vi "PH_ImageOperator.FF ConvexHull.vi"(0 "Image Src":T1, 5 "error in (no error)":errorcluster) -> (14 "Image Dst Out":T1, 19 "error out":errorcluster)   [LabVIEW 2014, in "PH_ImageOperator.lvlib"]
doc: "Calculate the convex hull of a given input image."
uses:
  PH_ImageOperator.lvlib
  <vilib>/vision/Image Controls.llb/IMAQ Image.ctl
  <vilib>/vision/NI_Vision_Development_Module.lvlib
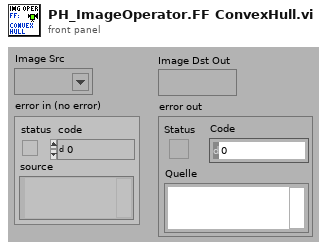
[diagram p1: front panel]
types:
  T1 = typedef "IMAQ Image.ctl" = refnum<image>
  T2 = cluster{"Area":dbl, "Number of Holes":dbl, "Bounding Rect":cluster{"Left":dbl, "Top":dbl, "Right":dbl, "Bottom":dbl}, "Center of Mass":cluster{"X":dbl, "Y":dbl}, "Orientation":dbl, "Dimensions":cluster{"Width":dbl, "Height":dbl}}[]
  T3 = typedef "Image Type" = u32
  T4 = cluster{"Area":dbl, "Number of Holes":dbl, "Bounding Rect":cluster{"Left":dbl, "Top":dbl, "Right":dbl, "Bottom":dbl}, "Center of Mass":cluster{"X":dbl, "Y":dbl}, "Orientation":dbl, "Dimensions":cluster{"Width":dbl, "Height":dbl}}
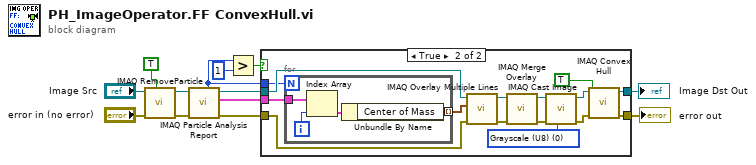
[diagram p0: block diagram]
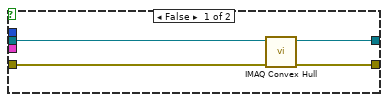
[diagram p2: hidden frame]
diagram:
  n1 = call "IMAQ RemoveParticle"("Square/Hexa (Square)"=TRUE, "error in (no error)"="error in (no error)", "Image Src"="Image Src") -> ("error out"=w8:errorcluster, "Image Dst Out"=w9:T1)  [unwired: 7 in]
  n2 = call "IMAQ Particle Analysis Report"("error in (no error)"=w8, "Image"=w9) -> ("error out"=w4:errorcluster, "Particle Reports (Pixels)"=w6:T2, "Image Out (duplicate)"=w10:T1, "Number of Particles"=w5:i32)  [unwired: 4 in, 2 out]
  n3 = Greater?(x=w5, y=1) -> (0:w7:bool)
  n4 = case shown="True" w7 {
    tunnel: [w14 w31] -> w13
    tunnel: w4 -> [w16 w27]
    tunnel: w10 -> [w17 w29]
    tunnel: [w15 w32] -> w12
    tunnel: w6 -> [_ w30]
    tunnel: w5 -> [_ w26]
    frame False {
      n5 = call "IMAQ Convex Hull"("error in (no error)"=w16, "Image Src"=w17) -> ("error out"=w14:errorcluster, "Image Dst Out"=w15:T1)  [unwired: 8 in]
    }
    frame True {
      w19 = T3 0 items=["Grayscale (U8)", "Grayscale (I16)", "Grayscale (SGL)", "Complex (CSG)", "RGB (U32)", "HSL (U32)", "RGB (U64)"] ("Image Type")
      n6 = for {
        N: w26 -> [_]
        tunnel: w30 -> [w36]
        tunnel: [w34] -> w28 mode=indexing
        i -> [w33]
        n7 = Index Array(array=w36, index=w33) -> (element=w35:T4)
        n8 = Unbundle By Name(w35) -> ("Center of Mass"=w34:cluster{"X":dbl, "Y":dbl})
      }
      n9 = call "IMAQ Overlay Multiple Lines"("error in (no error)"=w27, "Line End Points"=w28, "Image"=w29) -> ("error out"=w25:errorcluster, "Image Out"=w24:T1)  [unwired: 7 in]
      n10 = call "IMAQ Merge Overlay"("error in (no error)"=w25, "Image Src"=w24) -> ("error out"=w22:errorcluster, "Image Dst Out"=w23:T1)  [unwired: 8 in]
      n11 = call "IMAQ Cast Image"("Image Type"=w19, "error in (no error)"=w22, "Image Src"=w23) -> ("error out"=w20:errorcluster, "Image Dst Out"=w21:T1)  [unwired: 7 in]
      n12 = call "IMAQ Convex Hull"("error in (no error)"=w20, "Connectivity 4/8 (8)"=TRUE, "Image Src"=w21) -> ("error out"=w31:errorcluster, "Image Dst Out"=w32:T1)  [unwired: 7 in]
    }
  }
  "error out" <- w13
  "Image Dst Out" <- w12
